vi "Stop all Entities.vi"(8 "error in (no error)":errorcluster, 11 "Entity Table in":refnum<class "Entity Table.lvclass">) -> (0 "error out":errorcluster, 3 "Entity Table out":refnum<class "Entity Table.lvclass">)   [LabVIEW 2020, in "Entity Table.lvclass"]
doc: "Sends a Stop message to all Actors in the Entity Table."
uses:
  Entity Table.lvclass
  <vilib>/ActorFramework/Stop Msg/Stop Msg.lvclass
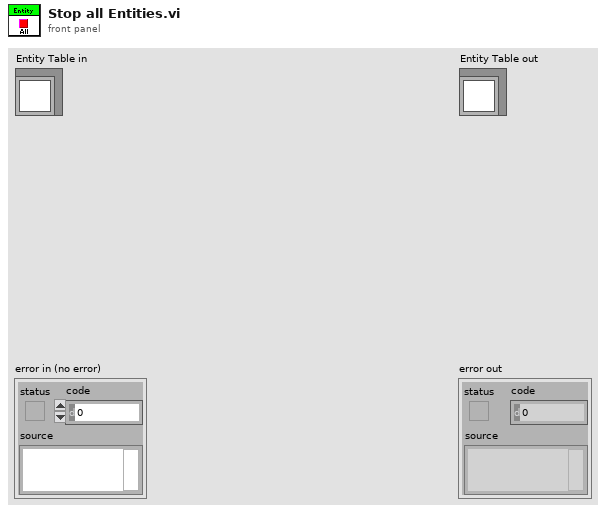
[diagram p1: front panel]
types:
  T1 = typedef "Entity Table.lvclass/Entity Table Element.ctl" = cluster{"Entity":refnum<class "Message Enqueuer.lvclass">[], "Entity Data":T2[]}
  T2 = typedef "Entity Table.lvclass/Entity Data.ctl" = cluster{"Name":string, "Status":string}
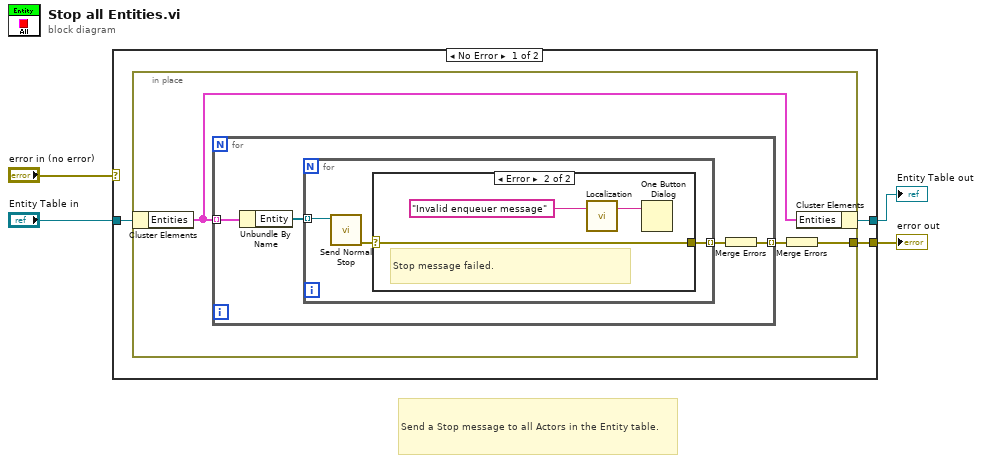
[diagram p0: block diagram]
diagram:
  # "Send a Stop message to all Actors in the Entity table."
  n1 = case shown="No Error" "error in (no error)" {
    selector: "error in (no error)" -> [_ w23]
    tunnel: [w6 w23] -> w3
    tunnel: [w5 w22] -> w1
    tunnel: "Entity Table in" -> [w7 w22]
    frame No Error {
      n2 = in-place "In Place Element Structure" {
        in-place-border: [w9] -> w6
        n3 = in-place-cluster #1 ("Unbundle / Bundle Elements")(w7) -> ("Entities"=w8:T1[])
        n4 = for {
          tunnel: w8 -> [w14] mode=indexing
          tunnel: [w11] -> w10 mode=indexing
          n5 = Unbundle By Name(w14) -> ("Entity"=w13:refnum<class "Message Enqueuer.lvclass">[])
          n6 = for {
            tunnel: w13 -> [w17] mode=indexing
            tunnel: [w15] -> w12 mode=indexing
            n7 = call <vilib>:"Send Normal Stop.vi"("Message Enqueuer"=w17) -> ("error out"=w16:errorcluster)  [unwired: 10 in]
            n8 = case shown="Error" w16 {
              selector: w16 -> [w18 w21]
              tunnel: [w18 w21] -> w15
              frame No Error {
                # "Stop message sent successfully."
              }
              frame Error {
                # "Stop message failed."
                n9 = call "Localization.vi"("untranslated"="Invalid enqueuer message" ("message")) -> ("translated"=w19:string)  [unwired: 2 in]
                n10 = One Button Dialog(message=w19) -> ()  [unwired: 1 in, 1 out]
              }
            }
          }
          n11 = Merge Errors(w12) -> (w11:errorcluster)
        }
        n12 = Merge Errors(w10) -> (w9:errorcluster)
        n13 = in-place-cluster #1 ("Unbundle / Bundle Elements")("Entities"=w8) -> (w5:refnum<class "Entity Table.lvclass">)
      }
    }
    frame Error {
    }
  }
  "error out" <- w3
  "Entity Table out" <- w1
